vi "Get system Hour&Min.vi"(8 "error in (no error)":errorcluster) -> (0 "error out":errorcluster, 1 "date/time string":string, 2 "minute":i32, 3 "hour":i32)   [LabVIEW 2014]
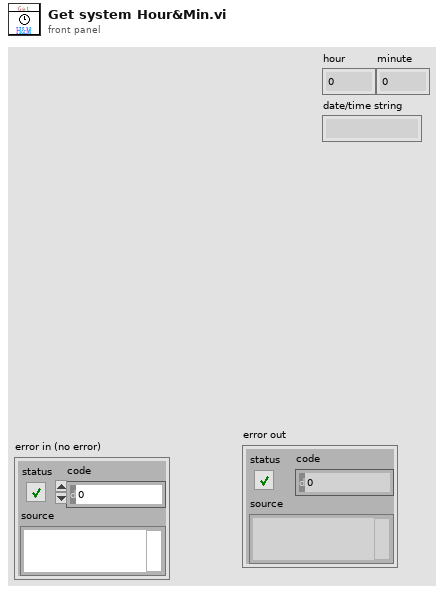
[diagram p1: front panel]
types:
  T1 = typedef "LVDateTimeRec.ctl" = cluster{"fractional second":dbl, "second":i32, "minute":i32, "hour":i32, "day of month":i32, "month":i32, "year":i32, "day of week":i32, "day of year":i32, "DST":i32}
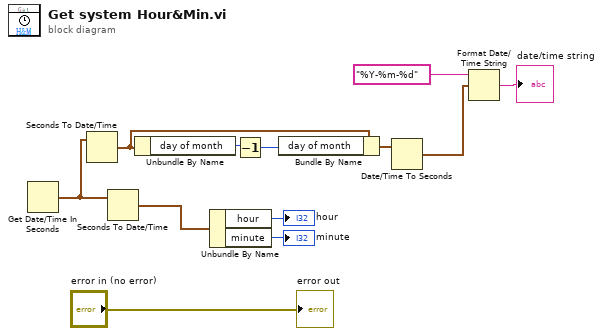
[diagram p0: block diagram]
diagram:
  n1 = Get Date/Time In Seconds() -> (seconds since 1Jan1904=w6:timestamp)
  n2 = Seconds To Date/Time(time stamp (now)=w6) -> (date time rec=w5:T1)  [unwired: 1 in]
  n3 = Seconds To Date/Time(time stamp (now)=w6) -> (date time rec=w12:T1)  [unwired: 1 in]
  n4 = Unbundle By Name(w5) -> ("day of month"=w4:i32)
  n5 = Unbundle By Name(w12) -> ("hour"=→"hour":i32, "minute"=→"minute":i32)
  n6 = Decrement(x=w4) -> (x-1=w3:i32)
  n7 = Bundle By Name(cluster=w5, "day of month"=w3) -> (w2:T1)
  n8 = Date/Time To Seconds(2:w2) -> (0:w1:timestamp)  [unwired: 1 in]
  n9 = Format Date/Time String(time format string (%c)="%Y-%m-%d", seconds (now)=w1) -> (date/time string=→"date/time string":string)  [unwired: 1 in]
  "error out" <- "error in (no error)"
